vi "Read Image File Directories and Tags from file.vi"(4 "error in":errorcluster, 7 "File":refnum<file>) -> (0 "error out":errorcluster, 1 "Tags for each IFD":cluster{"Tags":T1[]}[](array[cluster]), 2 "Litt/BigEnd":bool, 3 "File":refnum<file>)   [LabVIEW 2015, in "Tiff reader.lvlib"]
doc: "Reads the tags and associated data in a tiff file byte stream (Image Data in) starting at an offset (Image File Directory Offset) which is determined using the Read Header.vi. Returns an array of clusters containing the tag and location and format of the assocaited data."
uses:
  Tiff reader.lvlib
  FieldTypes.ctl
  IFD Entry.ctl
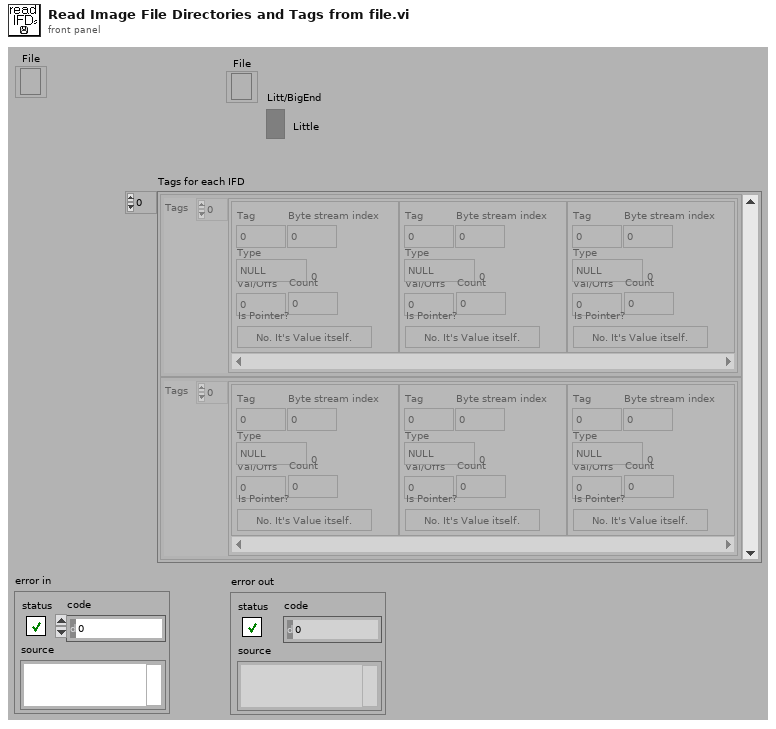
[diagram p1: front panel]
types:
  T1 = typedef "Tiff reader.lvlib/IFD Entry.ctl" = cluster{"Tag":u16, "Type":T2, "Count":u32, "Val/Offs":u32, "Is Pointer?":bool, "Byte stream index":i32}
  T2 = typedef "Tiff reader.lvlib/FieldTypes.ctl" = enum16{"NULL", "U8", "ASCII7", "U16", "U32", "RATIONAL", "SByte(I8)", "Undef(8Bit)", "I16", "I32", "SRat(4B:4B)", "SGL(4Byte)", "DBL(8Byte)"}
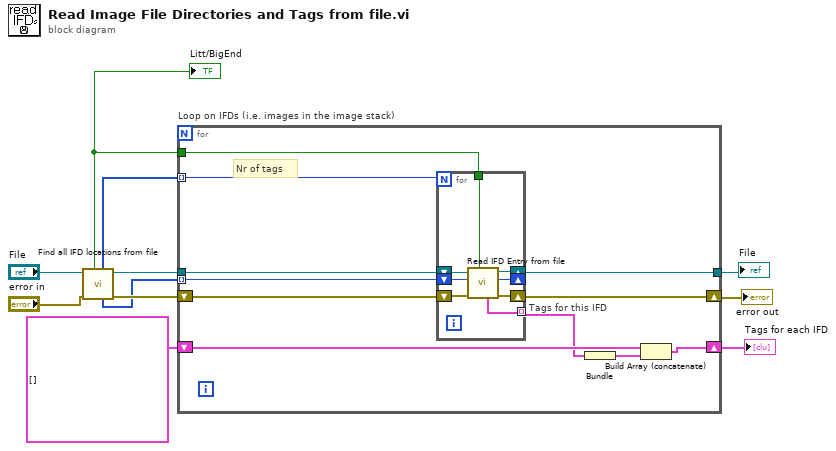
[diagram p0: block diagram]
diagram:
  n1 = call "Find all IFD locations from file.vi"("error in"="error in", "File"="File") -> ("error out"=w7:errorcluster, "File"=w8:refnum<file>, "1st tag locations"=w4:u32[], "# of tags in each IFD"=w6:u16[], "Litt/BigEnd"=w5:bool)  [unwired: 5 out]
  "Litt/BigEnd" <- w5
  n2 = for "Loop on IFDs (i.e. images in the image stack)" {
    tunnel: w8 -> [w14]
    tunnel: [w22] -> w10
    shift-right: [w20] -> w11
    shift-left: cluster{T1[]}[] [] -> [w21]
    tunnel: w5 -> [w19]
    shift-right: [w12] -> w2
    shift-left: w7 -> [w15]
    tunnel: w6 -> [w16] mode=indexing
    tunnel: w4 -> [w13] mode=indexing
    # "Tags for this IFD"
    # "Nr of tags"
    n3 = for {
      N: w16 -> [_]
      shift-right: [w25] -> w22
      shift-left: w14 -> [w30]
      shift-right: [w26] -> _
      shift-left: w13 -> [w27]
      tunnel: [w23] -> w17 mode=indexing
      tunnel: w19 -> [w24]
      shift-right: [w28] -> w12
      shift-left: w15 -> [w29]
      n4 = call "Read IFD Entry from file.vi"("Litt/BigEnd"=w24, "error in"=w29, "Tag location in"=w27, "File"=w30) -> ("error out"=w28:errorcluster, "Next Tag location Out\n(IN + 12)"=w26:i64, "File"=w25:refnum<file>, "Tag"=w23:T1)  [unwired: 1 in, 3 out]
    }
    n5 = Bundle(w17) -> (w18:cluster{T1[]})  [unwired: 1 in]
    n6 = Build Array (concatenate)(w21, w18) -> (w20:cluster{T1[]}[])
  }
  "File" <- w10
  "Tags for each IFD" <- w11
  "error out" <- w2
